vi "dattoimage.vi"(2 "image2list":u16, 3 "Current Average":sgl, 4 "image1list":u16) -> (0 "image 2 array out":sgl[][](array[numeric]), 1 "image 1 array out":sgl[][](array[numeric]))   [LabVIEW 2015]
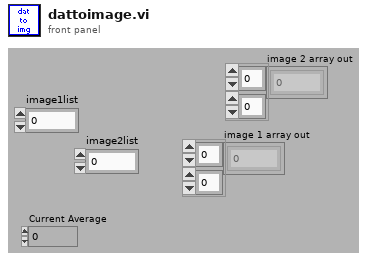
[diagram p1: front panel]
types:
  T1 = typedef "LVRectTypeDef.ctl" = cluster{"Left":i16, "Top":i16, "Right":i16, "Bottom":i16}
  T2 = cluster{"Xpixels":i32, "Vxminref":dbl, "Vxmaxref":dbl, "P":dbl, "Ypixels":i32, "Vyminref":dbl, "Vymaxref":dbl, "srate":sgl, "sAOxy":i32, "timeout":dbl, "type":string, "date":string, "time":string, "Colormap":u16, "Drawing Mode":u16, "Scanning Mode":u16, "square pixels":bool, "square matrix":bool, "Xpixels Img":i32, "Vx-min Img":dbl, "VX-max Img":dbl, "Ypixels Img":i32, "Vy-min Img":dbl, "Vy-max Img ":dbl, "Angle Img":dbl, "autoshutter":bool, "finite":bool, "cont":bool, "wavdet":bool, "measpoints":i32, "avpp":i32, "bufferAO":i32, "bufferAI":i32, "starttick":u32, "waveform":path, "Vx-ref":dbl, "Vy-ref":dbl, "refreshrate":dbl, "refreshbuffer":i32, "tt_cycles":i32, "motorref":refnum<k7>, "mirrorswitch":refnum<k7>, "sample mode":i32, "maxbufferAI":i32, "srateAODO":sgl, "bin":sgl, "Pel":sgl, "Angle draw":dbl, "srate Img":sgl, "ROIimg_plotbounds":T1, "auto OD":bool, "ODfilt":u16, "aAI":i32[], "aCI":i32[], "aAO":u32[], "aDO":u32[], "refwfsize":dbl, "Lifetime":bool, "Vz-Img":dbl, "Vz-ref":dbl, "Vz-reset":dbl, "AIoverride":bool}
  T3 = cluster{" AI":refnum<k21>, "E_AI":errorcluster, "header":dbl[]}
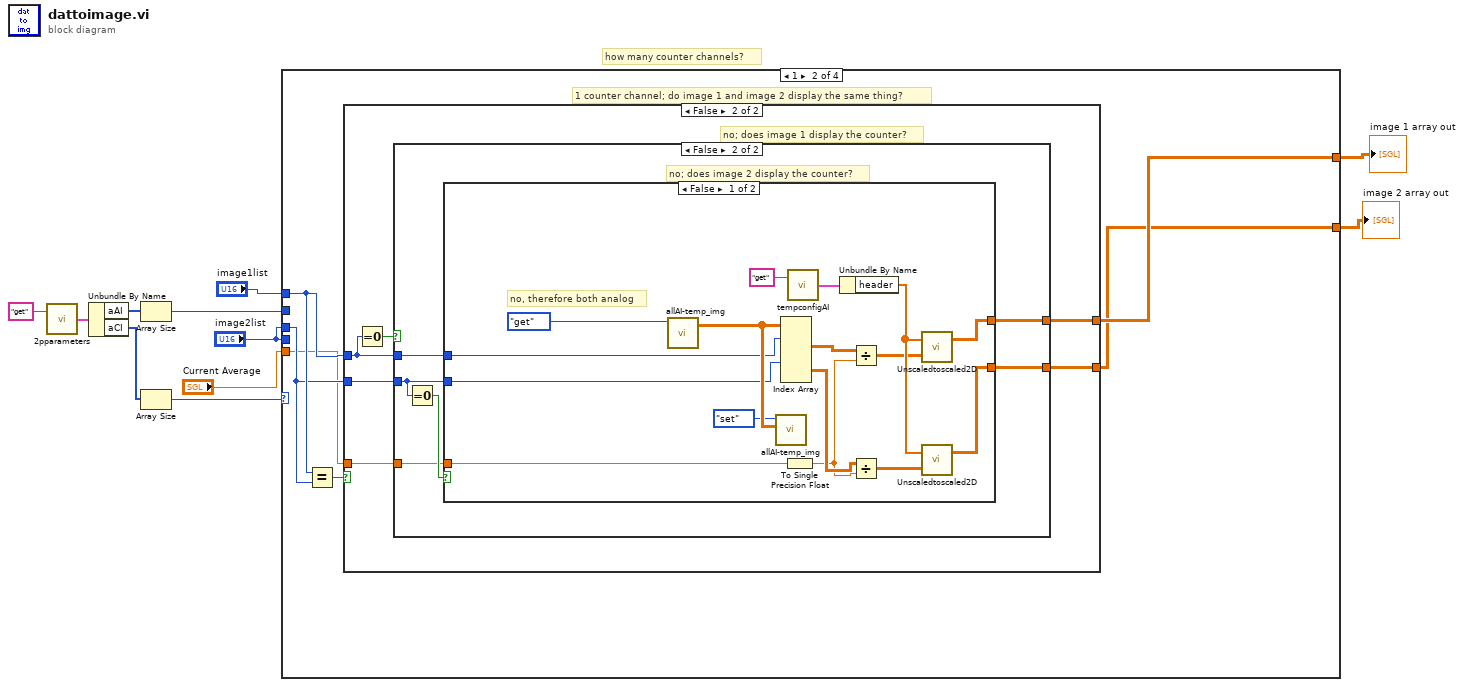
[diagram p0: block diagram]
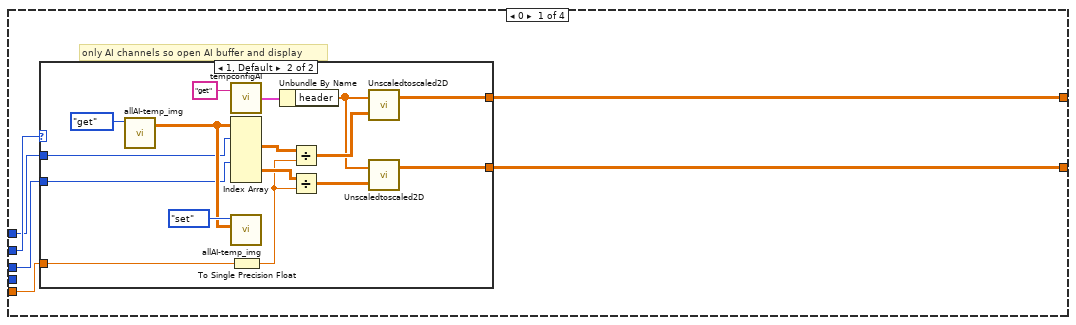
[diagram p2: hidden frame]
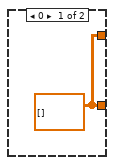
[diagram p3: hidden frame]
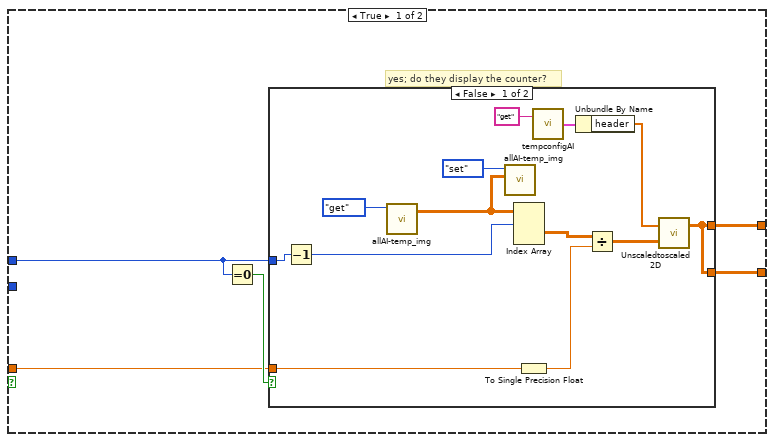
[diagram p4: hidden frame]
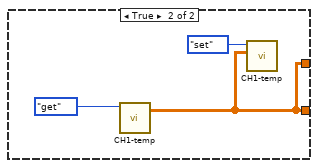
[diagram p5: hidden frame]
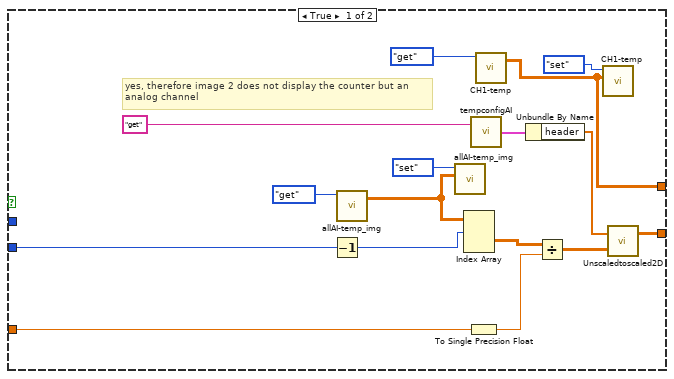
[diagram p6: hidden frame]
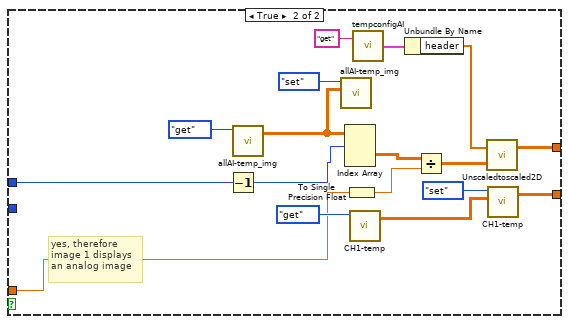
[diagram p7: hidden frame]
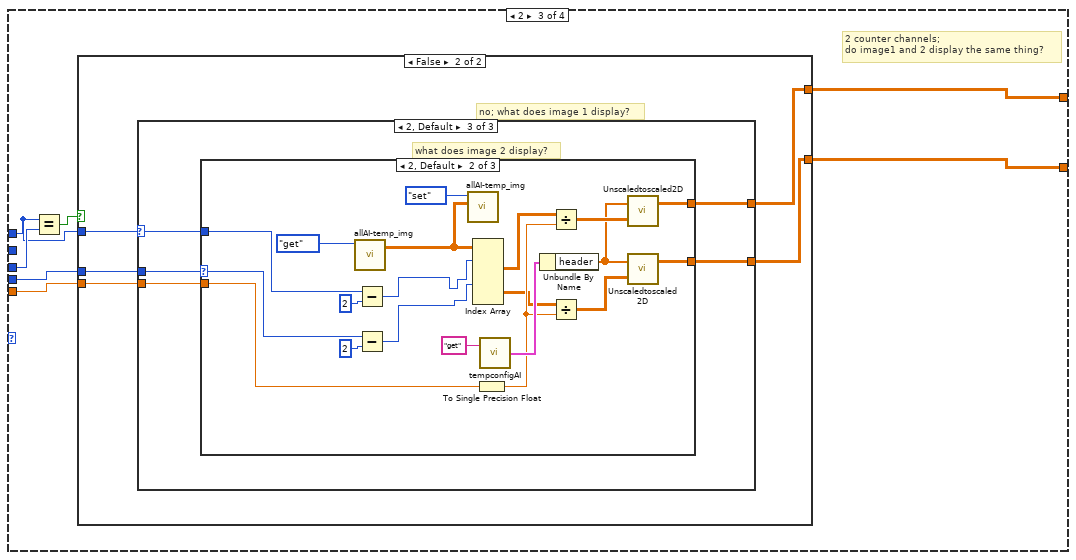
[diagram p8: hidden frame]
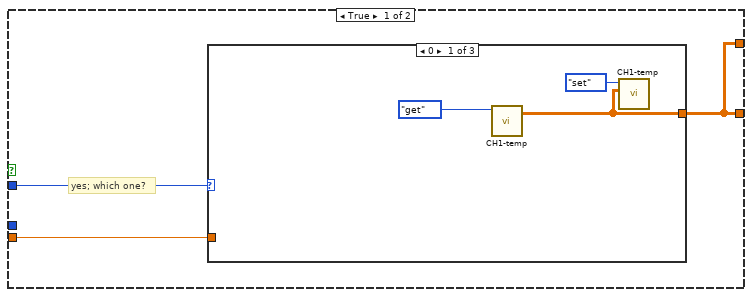
[diagram p9: hidden frame]
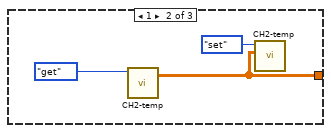
[diagram p10: hidden frame]
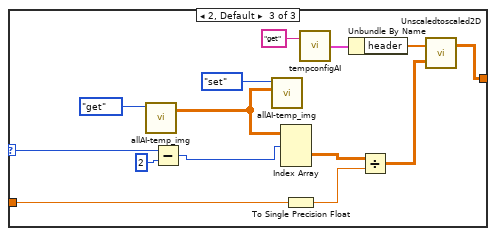
[diagram p11: hidden frame]
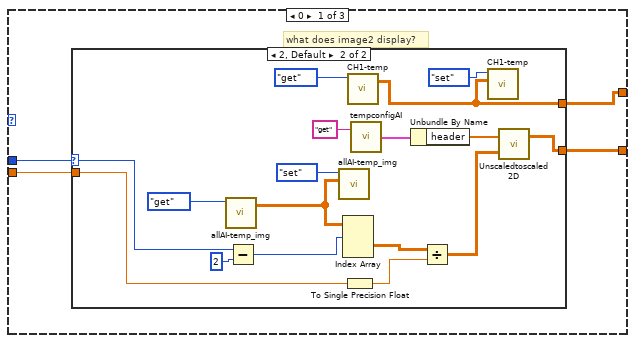
[diagram p12: hidden frame]
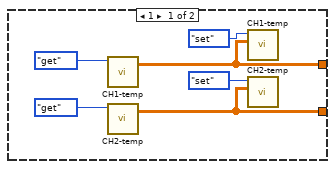
[diagram p13: hidden frame]
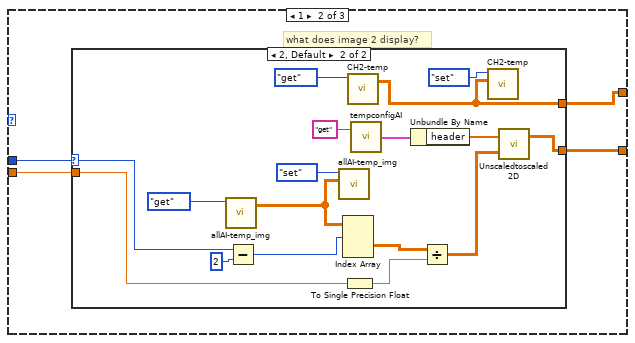
[diagram p14: hidden frame]
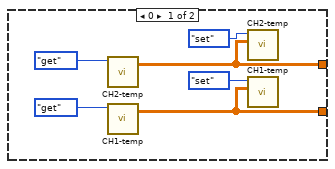
[diagram p15: hidden frame]
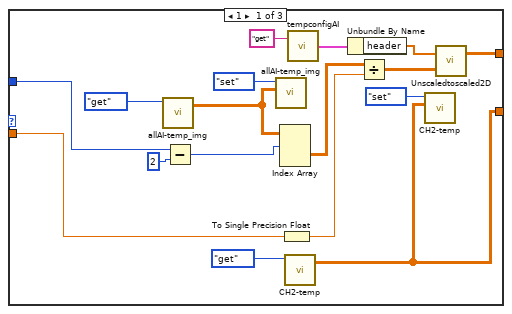
[diagram p16: hidden frame]
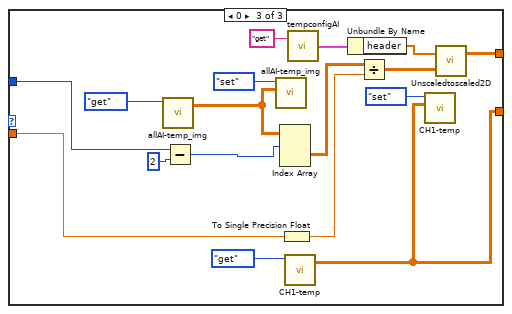
[diagram p17: hidden frame]
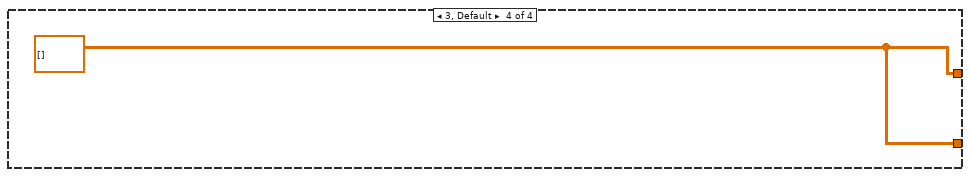
[diagram p18: hidden frame]
diagram:
  # "how many counter channels?"
  n1 = call "2pparameters.vi"("command"="get") -> ("params out"=w10:T2)  [unwired: 1 in]
  n2 = Unbundle By Name(w10) -> ("aAI"=w6:i32[], "aCI"=w9:i32[])
  n3 = Array Size(array=w6) -> (size(s)=w5:i32)
  n4 = Array Size(array=w9) -> (size(s)=w8:i32)
  n5 = case shown="1" w8 {
    tunnel: [w17 w40 w129 w271] -> w7
    tunnel: w5 -> [w16 _ _ _]
    tunnel: [w15 w37 w125 w271] -> w4
    tunnel: "image1list" -> [w14 w39 w126 _]
    tunnel: "image2list" -> [w13 w36 w128 _]
    tunnel: "image2list" -> [_ _ w124 _]
    tunnel: "Current Average" -> [w12 w35 w123 _]
    frame 0 {
      # "only AI channels so open AI buffer and display"
      n6 = case shown="1, Default" w16 {
        tunnel: [w18 w34] -> w17
        tunnel: [w18 w24] -> w15
        tunnel: w14 -> [_ w22]
        tunnel: w13 -> [_ w21]
        tunnel: w12 -> [_ w23]
        frame 0 {
          w18 = sgl[][] []
        }
        frame 1, Default {
          n7 = call "allAI-temp_img.vi"("command"=enum16{"get", "set", "clear", "append"}."get") -> ("array out"=w28:sgl[][][])  [unwired: 3 in, 1 out]
          n8 = call "tempconfigAI.vi"("command"="get") -> ("Temp Config out"=w32:T3)  [unwired: 1 in]
          n9 = Index Array(array=w28, index (dim 0) #1=w22, index (dim 0) #2=w21) -> (element #1=w29:sgl[][], element #2=w20:sgl[][])  [unwired: 4 in]
          n10 = call "allAI-temp_img.vi"("array in"=w28, "command"=enum16{"get", "set", "clear", "append"}."set") -> ()  [unwired: 2 in, 2 out]
          n11 = To Single Precision Float(number=w23) -> (single precision float=w19:sgl)
          n12 = Unbundle By Name(w32) -> ("header"=w26:dbl[])
          n13 = Divide(x=w29, y=w19) -> (x/y=w27:sgl[][])
          n14 = Divide(x=w20, y=w19) -> (x/y=w25:sgl[][])
          n15 = call "Unscaledtoscaled2D.vi"("Unscaled Data"=w27, "Header Information"=w26) -> ("Array"=w34:sgl[][])  [unwired: 1 in]
          n16 = call "Unscaledtoscaled2D.vi"("Unscaled Data"=w25, "Header Information"=w26) -> ("Array"=w24:sgl[][])  [unwired: 1 in]
        }
      }
    }
    frame 1 {
      # "1 counter channel; do image 1 and image 2 display the same thing?"
      n17 = Equal?(x=w39, y=w36) -> (x = y?=w38:bool)
      n18 = case shown="False" w38 {
        tunnel: [w45 w67] -> w40
        tunnel: w39 -> [w41 w63]
        tunnel: [w43 w65] -> w37
        tunnel: w36 -> [_ w64]
        tunnel: w35 -> [w42 w62]
        frame True {
          # "yes; do they display the counter?"
          n19 = Equal To 0?(x=w41) -> (x = 0?=w44:bool)
          n20 = case shown="False" w44 {
            tunnel: [w49 w59] -> w45
            tunnel: [w49 w59] -> w43
            tunnel: w42 -> [w48 _]
            tunnel: w41 -> [w47 _]
            frame False {
              n21 = Decrement(x=w47) -> (x-1=w46:u16)
              n22 = call "allAI-temp_img.vi"("command"=enum16{"get", "set", "clear", "append"}."get") -> ("array out"=w51:sgl[][][])  [unwired: 3 in, 1 out]
              n23 = call "allAI-temp_img.vi"("array in"=w51, "command"=enum16{"get", "set", "clear", "append"}."set") -> ()  [unwired: 2 in, 2 out]
              n24 = Index Array(array=w51, index (dim 0)=w46) -> (element=w53:sgl[][])  [unwired: 2 in]
              n25 = To Single Precision Float(number=w48) -> (single precision float=w52:sgl)
              n26 = call "tempconfigAI.vi"("command"="get") -> ("Temp Config out"=w57:T3)  [unwired: 1 in]
              n27 = Unbundle By Name(w57) -> ("header"=w56:dbl[])
              n28 = Divide(x=w53, y=w52) -> (x/y=w50:sgl[][])
              n29 = call "Unscaledtoscaled2D.vi"("Unscaled Data"=w50, "Header Information"=w56) -> ("Array"=w49:sgl[][])  [unwired: 1 in]
            }
            frame True {
              n30 = call "CH1-temp.vi"("command"=enum16{"get", "set", "clear", "add row"}."get") -> ("array out"=w59:sgl[][])  [unwired: 3 in, 1 out]
              n31 = call "CH1-temp.vi"("array in"=w59, "command"=enum16{"get", "set", "clear", "add row"}."set") -> ()  [unwired: 2 in, 2 out]
            }
          }
        }
        frame False {
          # "no; does image 1 display the counter?"
          n32 = Equal To 0?(x=w63) -> (x = 0?=w66:bool)
          n33 = case shown="False" w66 {
            tunnel: [w81 w88] -> w67
            tunnel: [w70 w87] -> w65
            tunnel: w64 -> [w72 w85]
            tunnel: w63 -> [_ w89]
            tunnel: w62 -> [w69 w84]
            frame True {
              # "yes, therefore image 2 does not display the counter but an\nanalog channel"
              n34 = Decrement(x=w72) -> (x-1=w68:u16)
              n35 = call "allAI-temp_img.vi"("command"=enum16{"get", "set", "clear", "append"}."get") -> ("array out"=w71:sgl[][][])  [unwired: 3 in, 1 out]
              n36 = call "allAI-temp_img.vi"("array in"=w71, "command"=enum16{"get", "set", "clear", "append"}."set") -> ()  [unwired: 2 in, 2 out]
              n37 = Index Array(array=w71, index (dim 0)=w68) -> (element=w75:sgl[][])  [unwired: 2 in]
              n38 = To Single Precision Float(number=w69) -> (single precision float=w74:sgl)
              n39 = call "tempconfigAI.vi"("command"="get") -> ("Temp Config out"=w79:T3)  [unwired: 1 in]
              n40 = call "CH1-temp.vi"("command"=enum16{"get", "set", "clear", "add row"}."get") -> ("array out"=w81:sgl[][])  [unwired: 3 in, 1 out]
              n41 = Unbundle By Name(w79) -> ("header"=w78:dbl[])
              n42 = Divide(x=w75, y=w74) -> (x/y=w73:sgl[][])
              n43 = call "CH1-temp.vi"("array in"=w81, "command"=enum16{"get", "set", "clear", "add row"}."set") -> ()  [unwired: 2 in, 2 out]
              n44 = call "Unscaledtoscaled2D.vi"("Unscaled Data"=w73, "Header Information"=w78) -> ("Array"=w70:sgl[][])  [unwired: 1 in]
            }
            frame False {
              # "no; does image 2 display the counter?"
              n45 = Equal To 0?(x=w85) -> (x = 0?=w86:bool)
              n46 = case shown="False" w86 {
                tunnel: w89 -> [w92 w110]
                tunnel: [w95 w109] -> w88
                tunnel: [w96 w108] -> w87
                tunnel: w85 -> [w93 _]
                tunnel: w84 -> [w94 w107]
                frame False {
                  # "no, therefore both analog"
                  n47 = call "allAI-temp_img.vi"("command"=enum16{"get", "set", "clear", "append"}."get") -> ("array out"=w102:sgl[][][])  [unwired: 3 in, 1 out]
                  n48 = call "allAI-temp_img.vi"("array in"=w102, "command"=enum16{"get", "set", "clear", "append"}."set") -> ()  [unwired: 2 in, 2 out]
                  n49 = Index Array(array=w102, index (dim 0) #1=w92, index (dim 0) #2=w93) -> (element #1=w101:sgl[][], element #2=w91:sgl[][])  [unwired: 4 in]
                  n50 = To Single Precision Float(number=w94) -> (single precision float=w90:sgl)
                  n51 = call "tempconfigAI.vi"("command"="get") -> ("Temp Config out"=w98:T3)  [unwired: 1 in]
                  n52 = Unbundle By Name(w98) -> ("header"=w104:dbl[])
                  n53 = Divide(x=w101, y=w90) -> (x/y=w103:sgl[][])
                  n54 = Divide(x=w91, y=w90) -> (x/y=w105:sgl[][])
                  n55 = call "Unscaledtoscaled2D.vi"("Unscaled Data"=w103, "Header Information"=w104) -> ("Array"=w95:sgl[][])  [unwired: 1 in]
                  n56 = call "Unscaledtoscaled2D.vi"("Unscaled Data"=w105, "Header Information"=w104) -> ("Array"=w96:sgl[][])  [unwired: 1 in]
                }
                frame True {
                  # "yes, therefore\nimage 1 displays \nan analog image"
                  n57 = Decrement(x=w110) -> (x-1=w106:u16)
                  n58 = call "allAI-temp_img.vi"("command"=enum16{"get", "set", "clear", "append"}."get") -> ("array out"=w111:sgl[][][])  [unwired: 3 in, 1 out]
                  n59 = call "allAI-temp_img.vi"("array in"=w111, "command"=enum16{"get", "set", "clear", "append"}."set") -> ()  [unwired: 2 in, 2 out]
                  n60 = Index Array(array=w111, index (dim 0)=w106) -> (element=w114:sgl[][])  [unwired: 2 in]
                  n61 = To Single Precision Float(number=w107) -> (single precision float=w113:sgl)
                  n62 = call "CH1-temp.vi"("command"=enum16{"get", "set", "clear", "add row"}."get") -> ("array out"=w120:sgl[][])  [unwired: 3 in, 1 out]
                  n63 = call "tempconfigAI.vi"("command"="get") -> ("Temp Config out"=w118:T3)  [unwired: 1 in]
                  n64 = Unbundle By Name(w118) -> ("header"=w117:dbl[])
                  n65 = Divide(x=w114, y=w113) -> (x/y=w112:sgl[][])
                  n66 = call "Unscaledtoscaled2D.vi"("Unscaled Data"=w112, "Header Information"=w117) -> ("Array"=w109:sgl[][])  [unwired: 1 in]
                  n67 = call "CH1-temp.vi"("array in"=w120, "command"=enum16{"get", "set", "clear", "add row"}."set") -> ("array out"=w108:sgl[][])  [unwired: 2 in, 1 out]
                }
              }
            }
          }
        }
      }
    }
    frame 2 {
      # "2 counter channels;\ndo image1 and 2 display the same thing?"
      n68 = Equal?(x=w126, y=w128) -> (x = y?=w127:bool)
      n69 = case shown="False" w127 {
        tunnel: [w131 w156] -> w129
        tunnel: w126 -> [w132 w157]
        tunnel: [w131 w154] -> w125
        tunnel: w124 -> [_ w155]
        tunnel: w123 -> [w130 w153]
        frame True {
          # "yes; which one?"
          n70 = case shown="0" w132 {
            selector: w132 -> [_ _ w141]
            tunnel: [w133 w136 w143] -> w131
            tunnel: w130 -> [_ _ w140]
            frame 0 {
              n71 = call "CH1-temp.vi"("command"=enum16{"get", "set", "clear", "add row"}."get") -> ("array out"=w133:sgl[][])  [unwired: 3 in, 1 out]
              n72 = call "CH1-temp.vi"("array in"=w133, "command"=enum16{"get", "set", "clear", "add row"}."set") -> ()  [unwired: 2 in, 2 out]
            }
            frame 1 {
              n73 = call "CH2-temp.vi"("command"=enum16{"get", "set", "clear", "add row"}."get") -> ("array out"=w136:sgl[][])  [unwired: 3 in, 1 out]
              n74 = call "CH2-temp.vi"("array in"=w136, "command"=enum16{"get", "set", "clear", "add row"}."set") -> ()  [unwired: 2 in, 2 out]
            }
            frame 2, Default {
              n75 = call "allAI-temp_img.vi"("command"=enum16{"get", "set", "clear", "append"}."get") -> ("array out"=w145:sgl[][][])  [unwired: 3 in, 1 out]
              n76 = Subtract(x=w141, y=2) -> (x-y=w139:i32)
              n77 = call "allAI-temp_img.vi"("array in"=w145, "command"=enum16{"get", "set", "clear", "append"}."set") -> ()  [unwired: 2 in, 2 out]
              n78 = Index Array(array=w145, index (dim 0)=w139) -> (element=w147:sgl[][])  [unwired: 2 in]
              n79 = To Single Precision Float(number=w140) -> (single precision float=w146:sgl)
              n80 = call "tempconfigAI.vi"("command"="get") -> ("Temp Config out"=w151:T3)  [unwired: 1 in]
              n81 = Unbundle By Name(w151) -> ("header"=w150:dbl[])
              n82 = Divide(x=w147, y=w146) -> (x/y=w144:sgl[][])
              n83 = call "Unscaledtoscaled2D.vi"("Unscaled Data"=w144, "Header Information"=w150) -> ("Array"=w143:sgl[][])  [unwired: 1 in]
            }
          }
        }
        frame False {
          # "no; what does image 1 display?"
          n84 = case shown="2, Default" w157 {
            selector: w157 -> [_ _ w215]
            tunnel: [w161 w188 w216] -> w156
            tunnel: w155 -> [w160 w187 w214]
            tunnel: [w159 w186 w213] -> w154
            tunnel: w153 -> [w158 w185 w212]
            frame 0 {
              # "what does image2 display?"
              n85 = case shown="2, Default" w160 {
                selector: w160 -> [_ w171]
                tunnel: [w165 w182] -> w161
                tunnel: [w162 w170] -> w159
                tunnel: w158 -> [_ w169]
                frame 1 {
                  n86 = call "CH1-temp.vi"("command"=enum16{"get", "set", "clear", "add row"}."get") -> ("array out"=w165:sgl[][])  [unwired: 3 in, 1 out]
                  n87 = call "CH2-temp.vi"("command"=enum16{"get", "set", "clear", "add row"}."get") -> ("array out"=w162:sgl[][])  [unwired: 3 in, 1 out]
                  n88 = call "CH1-temp.vi"("array in"=w165, "command"=enum16{"get", "set", "clear", "add row"}."set") -> ()  [unwired: 2 in, 2 out]
                  n89 = call "CH2-temp.vi"("array in"=w162, "command"=enum16{"get", "set", "clear", "add row"}."set") -> ()  [unwired: 2 in, 2 out]
                }
                frame 2, Default {
                  n90 = call "allAI-temp_img.vi"("command"=enum16{"get", "set", "clear", "append"}."get") -> ("array out"=w174:sgl[][][])  [unwired: 3 in, 1 out]
                  n91 = Subtract(x=w171, y=2) -> (x-y=w168:i32)
                  n92 = call "allAI-temp_img.vi"("array in"=w174, "command"=enum16{"get", "set", "clear", "append"}."set") -> ()  [unwired: 2 in, 2 out]
                  n93 = Index Array(array=w174, index (dim 0)=w168) -> (element=w176:sgl[][])  [unwired: 2 in]
                  n94 = To Single Precision Float(number=w169) -> (single precision float=w175:sgl)
                  n95 = call "CH1-temp.vi"("command"=enum16{"get", "set", "clear", "add row"}."get") -> ("array out"=w182:sgl[][])  [unwired: 3 in, 1 out]
                  n96 = call "tempconfigAI.vi"("command"="get") -> ("Temp Config out"=w180:T3)  [unwired: 1 in]
                  n97 = Unbundle By Name(w180) -> ("header"=w179:dbl[])
                  n98 = Divide(x=w176, y=w175) -> (x/y=w173:sgl[][])
                  n99 = call "CH1-temp.vi"("array in"=w182, "command"=enum16{"get", "set", "clear", "add row"}."set") -> ()  [unwired: 2 in, 2 out]
                  n100 = call "Unscaledtoscaled2D.vi"("Unscaled Data"=w173, "Header Information"=w179) -> ("Array"=w170:sgl[][])  [unwired: 1 in]
                }
              }
            }
            frame 1 {
              # "what does image 2 display?"
              n101 = case shown="2, Default" w187 {
                selector: w187 -> [_ w198]
                tunnel: [w189 w209] -> w188
                tunnel: [w192 w197] -> w186
                tunnel: w185 -> [_ w196]
                frame 0 {
                  n102 = call "CH2-temp.vi"("command"=enum16{"get", "set", "clear", "add row"}."get") -> ("array out"=w189:sgl[][])  [unwired: 3 in, 1 out]
                  n103 = call "CH1-temp.vi"("command"=enum16{"get", "set", "clear", "add row"}."get") -> ("array out"=w192:sgl[][])  [unwired: 3 in, 1 out]
                  n104 = call "CH2-temp.vi"("array in"=w189, "command"=enum16{"get", "set", "clear", "add row"}."set") -> ()  [unwired: 2 in, 2 out]
                  n105 = call "CH1-temp.vi"("array in"=w192, "command"=enum16{"get", "set", "clear", "add row"}."set") -> ()  [unwired: 2 in, 2 out]
                }
                frame 2, Default {
                  n106 = call "allAI-temp_img.vi"("command"=enum16{"get", "set", "clear", "append"}."get") -> ("array out"=w201:sgl[][][])  [unwired: 3 in, 1 out]
                  n107 = Subtract(x=w198, y=2) -> (x-y=w195:i32)
                  n108 = call "allAI-temp_img.vi"("array in"=w201, "command"=enum16{"get", "set", "clear", "append"}."set") -> ()  [unwired: 2 in, 2 out]
                  n109 = Index Array(array=w201, index (dim 0)=w195) -> (element=w203:sgl[][])  [unwired: 2 in]
                  n110 = To Single Precision Float(number=w196) -> (single precision float=w202:sgl)
                  n111 = call "CH2-temp.vi"("command"=enum16{"get", "set", "clear", "add row"}."get") -> ("array out"=w209:sgl[][])  [unwired: 3 in, 1 out]
                  n112 = call "tempconfigAI.vi"("command"="get") -> ("Temp Config out"=w207:T3)  [unwired: 1 in]
                  n113 = Unbundle By Name(w207) -> ("header"=w206:dbl[])
                  n114 = Divide(x=w203, y=w202) -> (x/y=w200:sgl[][])
                  n115 = call "CH2-temp.vi"("array in"=w209, "command"=enum16{"get", "set", "clear", "add row"}."set") -> ()  [unwired: 2 in, 2 out]
                  n116 = call "Unscaledtoscaled2D.vi"("Unscaled Data"=w200, "Header Information"=w206) -> ("Array"=w197:sgl[][])  [unwired: 1 in]
                }
              }
            }
            frame 2, Default {
              # "what does image 2 display?"
              n117 = case shown="2, Default" w214 {
                selector: w214 -> [_ w242 _]
                tunnel: [w224 w246 w261] -> w216
                tunnel: w215 -> [w222 w244 w259]
                tunnel: [w219 w237 w256] -> w213
                tunnel: w212 -> [w218 w236 w255]
                frame 1 {
                  n118 = call "allAI-temp_img.vi"("command"=enum16{"get", "set", "clear", "append"}."get") -> ("array out"=w226:sgl[][][])  [unwired: 3 in, 1 out]
                  n119 = Subtract(x=w222, y=2) -> (x-y=w217:i32)
                  n120 = call "allAI-temp_img.vi"("array in"=w226, "command"=enum16{"get", "set", "clear", "append"}."set") -> ()  [unwired: 2 in, 2 out]
                  n121 = Index Array(array=w226, index (dim 0)=w217) -> (element=w228:sgl[][])  [unwired: 2 in]
                  n122 = To Single Precision Float(number=w218) -> (single precision float=w227:sgl)
                  n123 = call "CH2-temp.vi"("command"=enum16{"get", "set", "clear", "add row"}."get") -> ("array out"=w219:sgl[][])  [unwired: 3 in, 1 out]
                  n124 = call "tempconfigAI.vi"("command"="get") -> ("Temp Config out"=w232:T3)  [unwired: 1 in]
                  n125 = Unbundle By Name(w232) -> ("header"=w231:dbl[])
                  n126 = Divide(x=w228, y=w227) -> (x/y=w225:sgl[][])
                  n127 = call "CH2-temp.vi"("array in"=w219, "command"=enum16{"get", "set", "clear", "add row"}."set") -> ()  [unwired: 2 in, 2 out]
                  n128 = call "Unscaledtoscaled2D.vi"("Unscaled Data"=w225, "Header Information"=w231) -> ("Array"=w224:sgl[][])  [unwired: 1 in]
                }
                frame 2, Default {
                  n129 = call "allAI-temp_img.vi"("command"=enum16{"get", "set", "clear", "append"}."get") -> ("array out"=w248:sgl[][][])  [unwired: 3 in, 1 out]
                  n130 = Subtract(x=w244, y=2) -> (x-y=w235:i32)
                  n131 = Subtract(x=w242, y=2) -> (x-y=w234:i32)
                  n132 = call "allAI-temp_img.vi"("array in"=w248, "command"=enum16{"get", "set", "clear", "append"}."set") -> ()  [unwired: 2 in, 2 out]
                  n133 = Index Array(array=w248, index (dim 0) #1=w235, index (dim 0) #2=w234) -> (element #1=w249:sgl[][], element #2=w240:sgl[][])  [unwired: 4 in]
                  n134 = To Single Precision Float(number=w236) -> (single precision float=w241:sgl)
                  n135 = call "tempconfigAI.vi"("command"="get") -> ("Temp Config out"=w252:T3)  [unwired: 1 in]
                  n136 = Unbundle By Name(w252) -> ("header"=w239:dbl[])
                  n137 = Divide(x=w249, y=w241) -> (x/y=w247:sgl[][])
                  n138 = Divide(x=w240, y=w241) -> (x/y=w238:sgl[][])
                  n139 = call "Unscaledtoscaled2D.vi"("Unscaled Data"=w247, "Header Information"=w239) -> ("Array"=w246:sgl[][])  [unwired: 1 in]
                  n140 = call "Unscaledtoscaled2D.vi"("Unscaled Data"=w238, "Header Information"=w239) -> ("Array"=w237:sgl[][])  [unwired: 1 in]
                }
                frame 0 {
                  n141 = call "allAI-temp_img.vi"("command"=enum16{"get", "set", "clear", "append"}."get") -> ("array out"=w263:sgl[][][])  [unwired: 3 in, 1 out]
                  n142 = Subtract(x=w259, y=2) -> (x-y=w254:i32)
                  n143 = call "allAI-temp_img.vi"("array in"=w263, "command"=enum16{"get", "set", "clear", "append"}."set") -> ()  [unwired: 2 in, 2 out]
                  n144 = Index Array(array=w263, index (dim 0)=w254) -> (element=w265:sgl[][])  [unwired: 2 in]
                  n145 = To Single Precision Float(number=w255) -> (single precision float=w264:sgl)
                  n146 = call "CH1-temp.vi"("command"=enum16{"get", "set", "clear", "add row"}."get") -> ("array out"=w256:sgl[][])  [unwired: 3 in, 1 out]
                  n147 = call "tempconfigAI.vi"("command"="get") -> ("Temp Config out"=w269:T3)  [unwired: 1 in]
                  n148 = Unbundle By Name(w269) -> ("header"=w268:dbl[])
                  n149 = Divide(x=w265, y=w264) -> (x/y=w262:sgl[][])
                  n150 = call "CH1-temp.vi"("array in"=w256, "command"=enum16{"get", "set", "clear", "add row"}."set") -> ()  [unwired: 2 in, 2 out]
                  n151 = call "Unscaledtoscaled2D.vi"("Unscaled Data"=w262, "Header Information"=w268) -> ("Array"=w261:sgl[][])  [unwired: 1 in]
                }
              }
            }
          }
        }
      }
    }
    frame 3, Default {
      w271 = sgl[][] []
    }
  }
  "image 1 array out" <- w7
  "image 2 array out" <- w4
